vi "Write Cross Val.vi"(4 "Col Header Val 2":string, 6 "Col Header Name 2":string, 7 "Section Name":string, 8 "error in (no error)":errorcluster, 9 "Col Header Val 1":string, 10 "Col Header Name 1":string, 11 "Config Data":T1(array[cluster])) -> (0 "error out":errorcluster, 1 "Find?":bool, 3 "Config Data dup":T1(array[cluster]))   [LabVIEW 2020, in "GUCalibration2.lvlib"]
uses:
  GUCalibration2.lvlib
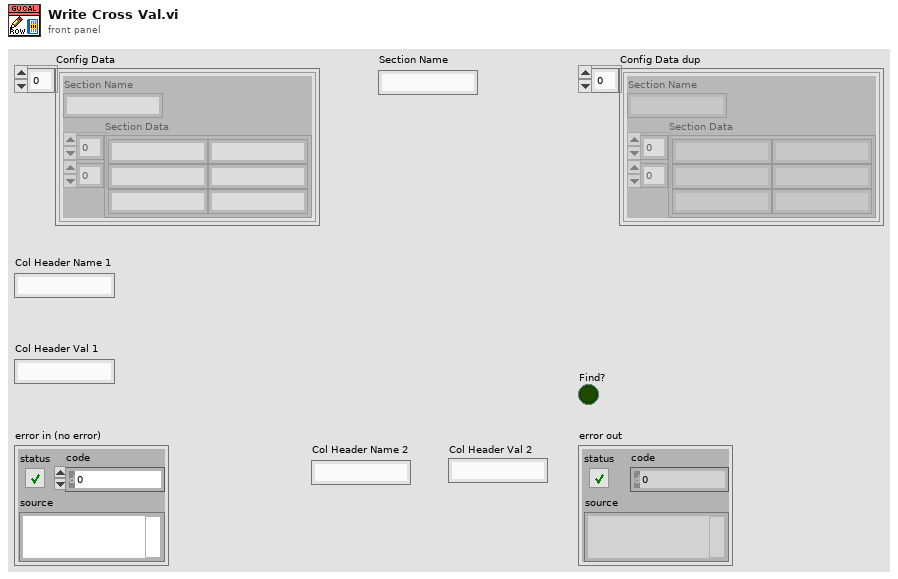
[diagram p1: front panel]
types:
  T1 = cluster{"Section Name":string, "Section Data":string[][]}[]
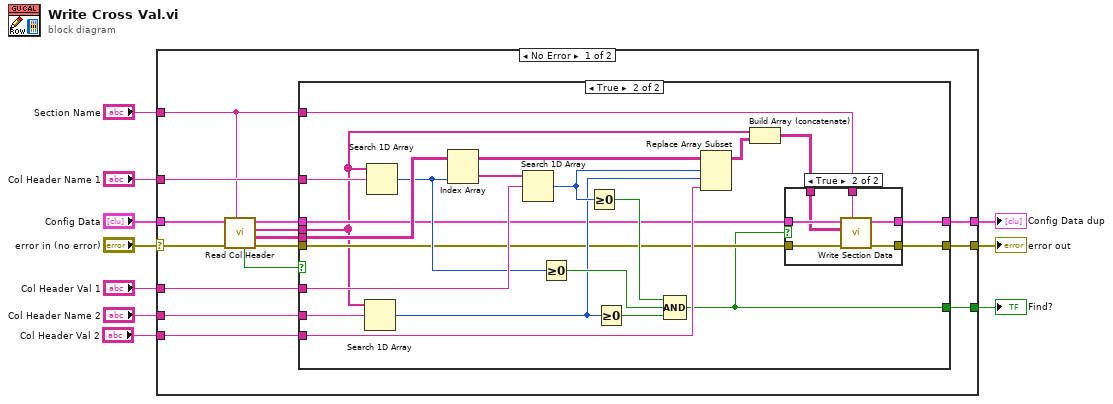
[diagram p0: block diagram]
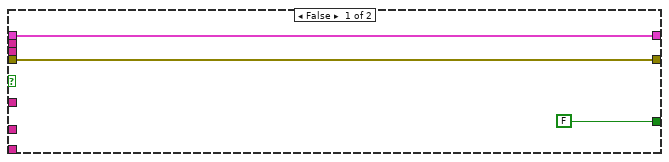
[diagram p2: hidden frame]
diagram:
  n1 = case shown="No Error" "error in (no error)" {
    selector: "error in (no error)" -> [w24 w59]
    tunnel: "Section Name" -> [w14 _]
    tunnel: "Config Data" -> [w25 w58]
    tunnel: [w17 w59] -> w7
    tunnel: [w15 w58] -> w6
    tunnel: [w12 _] -> w5
    tunnel: "Col Header Name 1" -> [w23 _]
    tunnel: "Col Header Val 1" -> [w22 _]
    tunnel: "Col Header Name 2" -> [w20 _]
    tunnel: "Col Header Val 2" -> [w19 _]
    frame No Error {
      n2 = call "Read Col Header.vi"("Section Name"=w14, "error in (no error)"=w24, "Config Data"=w25) -> ("error out"=w18:errorcluster, "Data"=w21:string[][], "Column Header"=w13:string[], "Config Data dup"=w16:T1, "Section Find?"=w11:bool)  [unwired: 4 in]
      n3 = case shown="True" w11 {
        tunnel: w23 -> [_ w49]
        tunnel: w22 -> [_ w46]
        tunnel: w21 -> [_ w44]
        tunnel: w20 -> [_ w41]
        tunnel: w19 -> [_ w38]
        tunnel: w18 -> [w27 w37]
        tunnel: [w27 w36] -> w17
        tunnel: w16 -> [w28 w35]
        tunnel: [w28 w34] -> w15
        tunnel: w14 -> [_ w33]
        tunnel: w13 -> [_ w32]
        tunnel: [FALSE w29] -> w12
        frame False {
        }
        frame True {
          n4 = Search 1D Array(1D array=w32, element=w41) -> (index of element=w39:i32)  [unwired: 1 in]
          n5 = Search 1D Array(1D array=w32, element=w49) -> (index of element=w42:i32)  [unwired: 1 in]
          n6 = Index Array(array=w44, index (col)=w42) -> (element=w47:string[])  [unwired: 1 in]
          n7 = Search 1D Array(1D array=w47, element=w46) -> (index of element=w43:i32)  [unwired: 1 in]
          n8 = Greater Or Equal To 0?(x=w42) -> (x >= 0?=w48:bool)
          n9 = Greater Or Equal To 0?(x=w43) -> (x >= 0?=w45:bool)
          n10 = Greater Or Equal To 0?(x=w39) -> (x >= 0?=w40:bool)
          n11 = Compound Arithmetic op=AND(w45, w48, w40) -> (w29:bool)
          n12 = Replace Array Subset(array=w44, new element=w38, index (row)=w43, index (col)=w39) -> (w31:string[][])
          n13 = Build Array (concatenate)(w32, w31) -> (w30:string[][])
          n14 = case shown="True" w29 {
            tunnel: w37 -> [w50 w57]
            tunnel: [w50 w56] -> w36
            tunnel: w35 -> [w51 w55]
            tunnel: [w51 w54] -> w34
            tunnel: w33 -> [_ w53]
            tunnel: w30 -> [_ w52]
            frame False {
            }
            frame True {
              n15 = call "Write Section Data.vi"("Section Name"=w53, "error in (no error)"=w57, "Section Data"=w52, "Config Data"=w55) -> ("error out"=w56:errorcluster, "Config Data out"=w54:T1)  [unwired: 6 in]
            }
          }
        }
      }
    }
    frame Error {
    }
  }
  "error out" <- w7
  "Config Data dup" <- w6
  "Find?" <- w5
